vi "Mix Samples.vi"(8 "error in (no error)":errorcluster, 11 "Samples In":refnum<class "Sample.lvclass">[](array[class])) -> (0 "error out":errorcluster, 1 "is clean?":bool, 2 "Empty Samples present?":bool, 3 "Sample out":refnum<class "Sample.lvclass">)   [LabVIEW 2015, in "Sample.lvclass"]
uses:
  Sample.lvclass
  Sample.lvclass/Sample.ctl
  Mixed Sample.vi
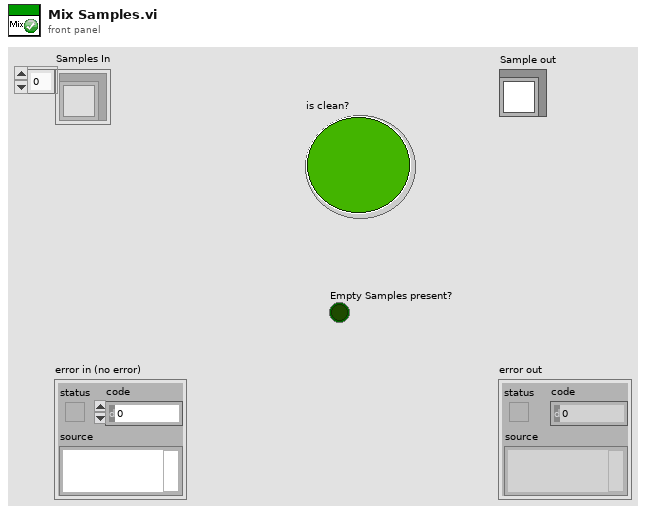
[diagram p1: front panel]
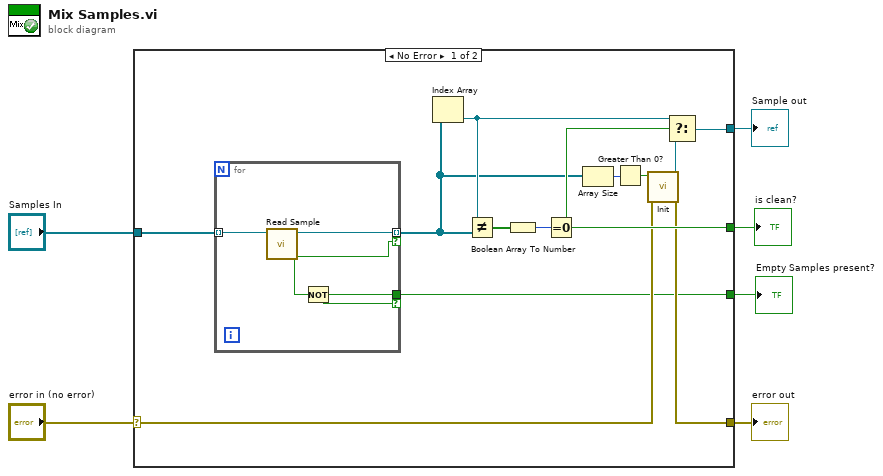
[diagram p0: block diagram]
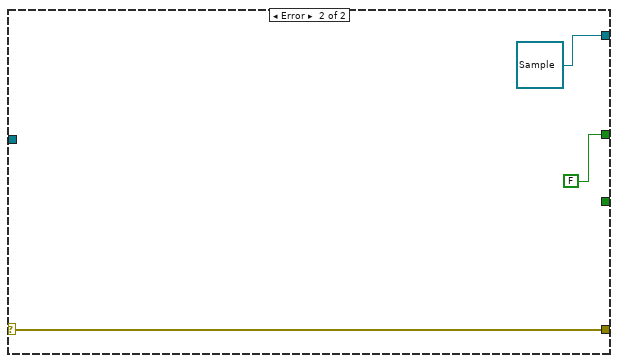
[diagram p2: hidden frame]
diagram:
  n1 = case shown="No Error" "error in (no error)" {
    selector: "error in (no error)" -> [w13 w26]
    tunnel: [w12 w26] -> w5
    tunnel: [w17 refnum<class "Sample.lvclass"> refnum ("Sample in")] -> w3
    tunnel: "Samples In" -> [w9 _]
    tunnel: [w15 FALSE] -> w2
    tunnel: [w7 _] -> w1
    frame No Error {
      n2 = for {
        tunnel: w9 -> [w23] mode=indexing
        tunnel: [w22] -> w8 mode=indexing if=w21
        tunnel: [w20] -> w7 if=w20
        n3 = call "Read Sample.vi"("Sample in"=w23) -> ("Sample In"=w21:bool, "Sample out"=w22:refnum<class "Sample.lvclass">)  [unwired: 6 in, 3 out]
        n4 = Not(x=w21) -> (.not. x?=w20:bool)
      }
      n5 = Index Array(array=w8) -> (element=w16:refnum<class "Sample.lvclass">)  [unwired: 1 in]
      n6 = Not Equal?(x=w16, y=w8) -> (x != y?=w19:bool[])
      n7 = Boolean Array To Number(Boolean array=w19) -> (number=w18:u32)
      n8 = Equal To 0?(x=w18) -> (x = 0?=w15:bool)
      n9 = Array Size(array=w8) -> (size(s)=w11:i32)
      n10 = Greater Than 0?(x=w11) -> (x > 0?=w10:bool)
      n11 = call "Init.vi"("error in (no error)"=w13, "Sample in"=w10) -> ("error out"=w12:errorcluster, "Sample out"=w14:refnum<class "Sample.lvclass">)  [unwired: 8 in]
      n12 = Select(t=w16, s=w15, f=w14) -> (s? t:f=w17:refnum<class "Sample.lvclass">)
    }
    frame Error {
    }
  }
  "error out" <- w5
  "Sample out" <- w3
  "is clean?" <- w2
  "Empty Samples present?" <- w1
